vi "Run.vi"(7 "Stop Demo":refnum<user-event>, 8 "error in":errorcluster, 9 "Try It Button":refnum<vi>, 10 "Main Subpanel":refnum<vi>, 11 "Demo in":refnum<class "Demo.lvclass">) -> (0 "error out":errorcluster, 3 "Demo out":refnum<class "Demo.lvclass">)   [LabVIEW 2020, in "Demo.lvclass"]
uses:
  Demo.lvclass
  Demo.lvclass/Demo.ctl
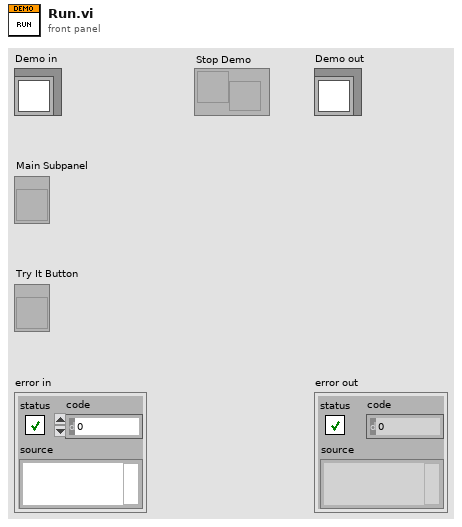
[diagram p1: front panel]
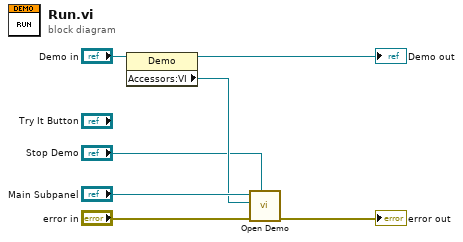
[diagram p0: block diagram]
diagram:
  n1 = property class="Demo"(reference="Demo in") -> (reference out=→"Demo out":refnum<class "Demo.lvclass">, "Accessors:VI"=w2:refnum<vi>)  [unwired: 1 in, 1 out]
  n2 = call "Open Demo.vi"("Stop Demo"="Stop Demo", "error in"="error in", "VI"=w2, "Main Subpanel"="Main Subpanel") -> ("error out"=→"error out":errorcluster)  [unwired: 7 in]
